vi "Set Laser Power.vi"(8 "error in (no error)":errorcluster, 9 "Power":dbl, 10 "Wavelength":u16, 11 "Laser Quantum in":refnum<class "Laser.lvclass">) -> (0 "error out":errorcluster, 3 "Laser Quantum out":refnum<class "Laser.lvclass">)   [LabVIEW 2018, in "Laser.lvlib" / "Laser.lvclass"]
uses:
  Laser.lvclass
  Laser.lvclass/Laser.ctl
  Resources/GLOBAL/GLOBAL Debug.vi
  Laser.lvlib
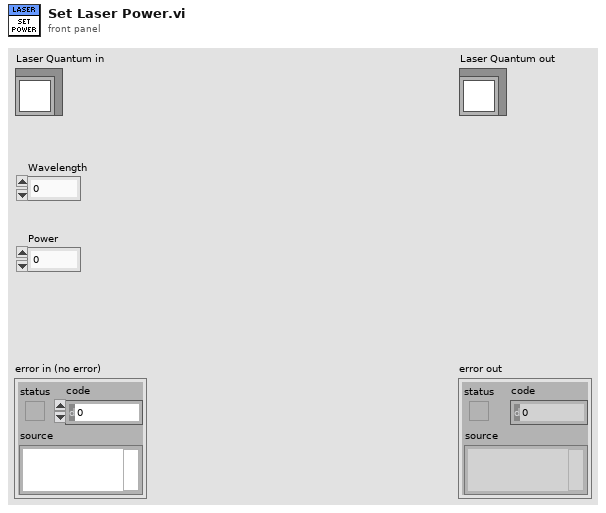
[diagram p1: front panel]
types:
  T1 = enum16{"Disable", "Laser Quantum", "Coherent OBIS", "PRM1-Z8", "Coherent HOPS"}
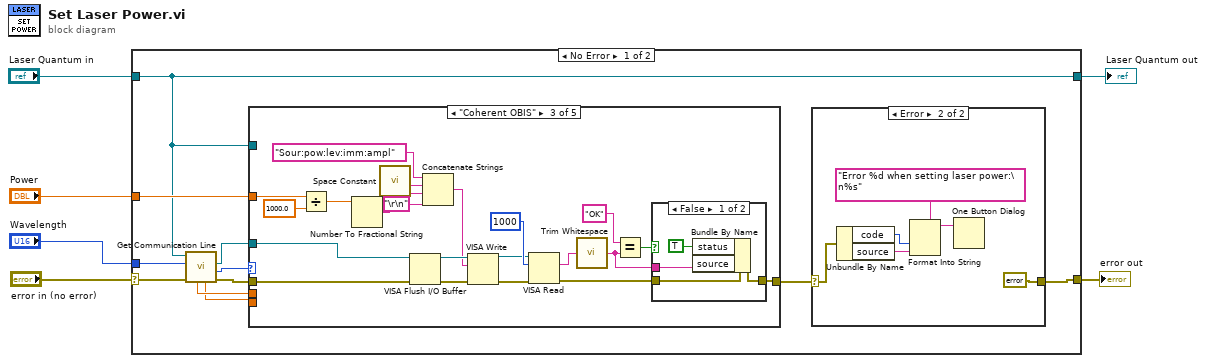
[diagram p0: block diagram]
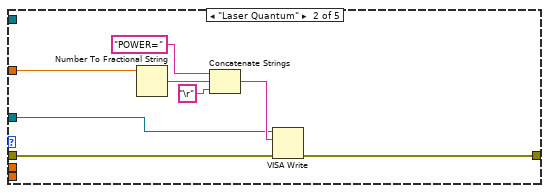
[diagram p3: hidden frame]
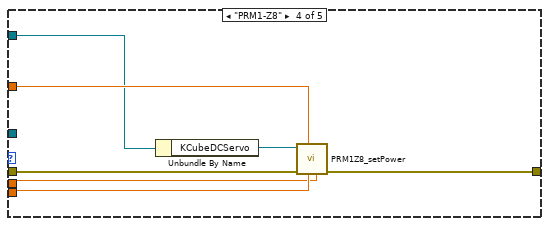
[diagram p5: hidden frame]
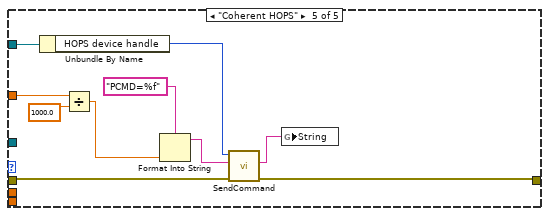
[diagram p6: hidden frame]
diagram:
  n1 = case shown="No Error" "error in (no error)" {
    selector: "error in (no error)" -> [w16 w78]
    tunnel: [w9 w78] -> w5
    tunnel: [w8 w77] -> w3
    tunnel: "Laser Quantum in" -> [w8 w77]
    tunnel: "Wavelength" -> [w7 _]
    tunnel: "Power" -> [w17 _]
    frame No Error {
      n2 = call-dynamic "Get Communication Line.vi"("error in (no error)"=w16, "Wavelength"=w7, "Laser Quantum in"=w8) -> ("error out"=w15:errorcluster, "Laser Type"=w13:T1, "Serial Port"=w14:refnum<visa-resource-name>, "Polarizer Theta Zero"=w11:dbl, "Polarizer Amplitude"=w12:dbl)  [unwired: 3 in, 1 out]
      n3 = case shown="\"Coherent OBIS\"" w13 {
        tunnel: w15 -> [w18 w20 w37 w56 w67]
        tunnel: w17 -> [_ w26 w38 w57 w65]
        tunnel: [w18 w22 w29 w59 w68] -> w10
        tunnel: w14 -> [_ w19 w36 _ _]
        tunnel: w12 -> [_ _ _ w55 _]
        tunnel: w11 -> [_ _ _ w54 _]
        tunnel: w8 -> [_ _ _ w53 w69]
        frame "Disable", Default {
        }
        frame "Laser Quantum" {
          n4 = Number To Fractional String(number=w26) -> (F-format string=w24:string)  [unwired: 3 in]
          n5 = Concatenate Strings("POWER=" ("write buffer"), w24, "\r" ("string")) -> (w23:string)
          n6 = VISA Write(VISA resource name=w19, write buffer=w23, error in (no error)=w20) -> (error out=w22:errorcluster)  [unwired: 2 out]
        }
        frame "Coherent OBIS" {
          n7 = Divide(x=w38, y=1000.0) -> (x/y=w43:dbl)
          n8 = Number To Fractional String(number=w43) -> (F-format string=w45:string)  [unwired: 3 in]
          n9 = call <vilib>:"Space Constant.vi"() -> ("String"=w44:string)
          n10 = VISA Flush I/O Buffer(VISA resource name=w36, error in (no error)=w37) -> (VISA resource name out=w46:refnum<visa-resource-name>, error out=w47:errorcluster)  [unwired: 1 in]
          n11 = Concatenate Strings("Sour:pow:lev:imm:ampl" ("write buffer"), w44, w45, "\r\n") -> (w42:string)
          n12 = VISA Write(VISA resource name=w46, write buffer=w42, error in (no error)=w47) -> (VISA resource name out=w33:refnum<visa-resource-name>, error out=w34:errorcluster)  [unwired: 1 out]
          n13 = VISA Read(VISA resource name=w33, byte count=u32 1000, error in (no error)=w34) -> (read buffer=w32:string, error out=w30:errorcluster)  [unwired: 2 out]
          n14 = call <vilib>:"Trim Whitespace.vi"("string"=w32) -> ("trimmed string"=w27:string)  [unwired: 1 in]
          n15 = Equal?(x="OK", y=w27) -> (x = y?=w28:bool)
          n16 = case shown="False" w28 {
            tunnel: w30 -> [w50 w52]
            tunnel: [w51 w52] -> w29
            tunnel: w27 -> [w49 _]
            frame False {
              n17 = Bundle By Name(cluster=w50, "status"=TRUE, "source"=w49) -> (w51:errorcluster)
            }
            frame True {
            }
          }
        }
        frame "PRM1-Z8" {
          n18 = Unbundle By Name(w53) -> ("KCubeDCServo"=w58:refnum<k24>)
          n19 = call "PRM1Z8_setPower.vi"("zero angle"=w54, "max power"=w55, "Target Power"=w57, "error in (no error)"=w56, "reference"=w58) -> ("error out"=w59:errorcluster)  [unwired: 5 in, 1 out]
        }
        frame "Coherent HOPS" {
          n20 = Unbundle By Name(w69) -> ("HOPS device handle"=w66:u64)
          n21 = Divide(x=w65, y=1000.0) -> (x/y=w62:dbl)
          n22 = Format Into String(format string="PCMD=%f" ("Command"), w62) -> (resulting string=w61:string)  [unwired: 2 in, 1 out]
          n23 = call "SendCommand.vi"("error in"=w67, "Command"=w61, "Device Handle"=w66) -> ("error out"=w68:errorcluster, "String"=w60:string)  [unwired: 3 in, 2 out]
          n24 = global write "GLOBAL Debug.vi" "String"(w60) -> ()
        }
      }
      n25 = case shown="Error" w10 {
        selector: w10 -> [w70 w71]
        tunnel: [w70 errorcluster {"status"=FALSE, "code"=0, "source"=""} ("error IO")] -> w9
        frame No Error {
        }
        frame Error {
          n26 = Unbundle By Name(w71) -> ("code"=w72:i32, "source"=w73:string)
          n27 = Format Into String(format string="Error %d when setting laser power:\n%s" ("message"), w72, w73) -> (resulting string=w75:string)  [unwired: 2 in, 1 out]
          n28 = One Button Dialog(message=w75) -> ()  [unwired: 1 in, 1 out]
        }
      }
    }
    frame Error {
    }
  }
  "error out" <- w5
  "Laser Quantum out" <- w3
